vi "Download zip file.vi"(0 "client handle":T1, 5 "Artifactory ZIP Directory":string, 7 "Zip File":string, 9 "Save Path":path=path "C:/Automation/APLs", 11 "Error In":errorcluster) -> (4 "client handle out":T1, 8 "Output Path":path, 10 "file or folder exists?":bool, 15 "Error Out":errorcluster)   [LabVIEW 2016]
uses:
  <vilib>/httpClient/ClientHandle.ctl
  <vilib>/regexp/Match Regular Expression.xnode
  <vilib>/httpClient/LabVIEWHTTPClient.lvlib
  <vilib>/zip/NI_Unzip.lvlib
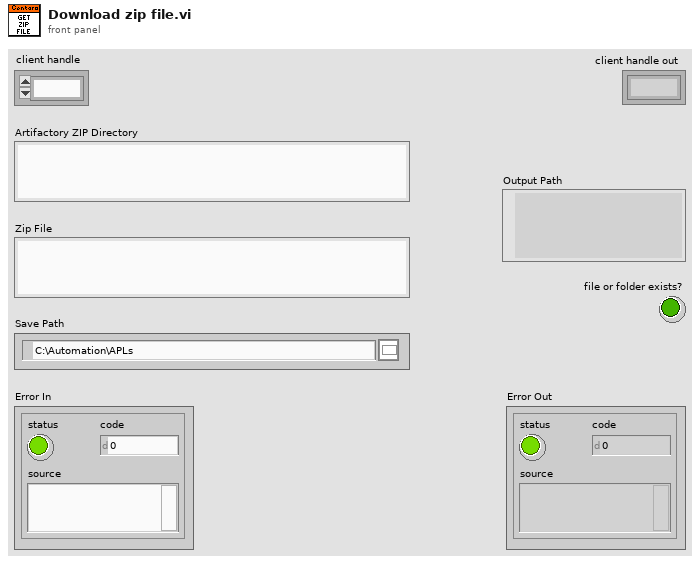
[diagram p1: front panel]
types:
  T1 = typedef "LabVIEWHTTPClient.lvlib/ClientHandle.ctl" = refnum<k1>
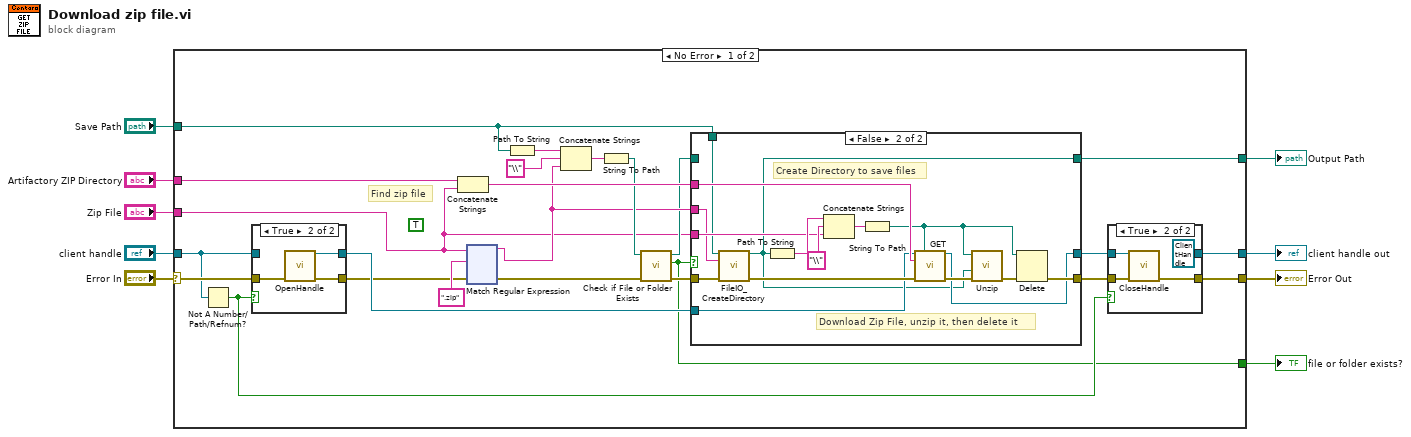
[diagram p0: block diagram]
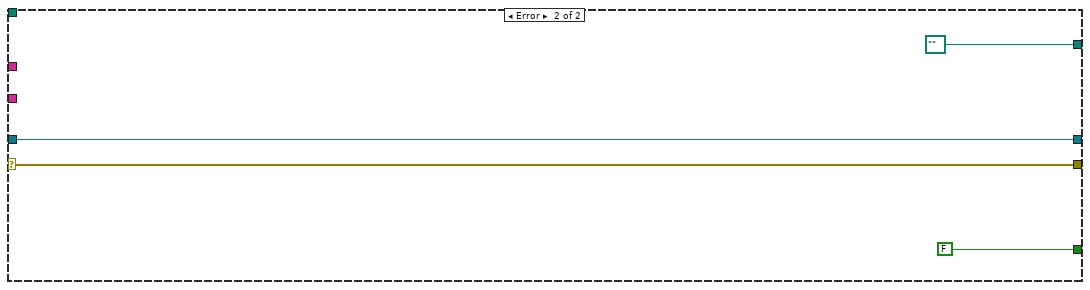
[diagram p5: hidden frame]
diagram:
  n1 = case shown="No Error" "Error In" {
    selector: "Error In" -> [w31 w181]
    tunnel: "client handle" -> [w24 w180]
    tunnel: [w33 w180] -> w8
    tunnel: [w32 w181] -> w7
    tunnel: "Artifactory ZIP Directory" -> [w28 _]
    tunnel: [w25 path ""] -> w4
    tunnel: "Save Path" -> [w21 _]
    tunnel: "Zip File" -> [w11 _]
    tunnel: [w13 FALSE ("file or folder exists?")] -> w1
    frame No Error {
      (unwired) TRUE ("multiline? (F)")
      # "Find zip file"
      n2 = Not A Number/Path/Refnum?(number/path/refnum=w24) -> (NaN/Path/Refnum?=w23:bool)
      n3 = case shown="True" w23 {
        tunnel: [w174 w177] -> w22
        tunnel: w24 -> [w174 _]
        tunnel: w31 -> [w173 w176]
        tunnel: [w173 w175] -> w10
        frame False {
        }
        frame True {
          n4 = call <vilib>:"OpenHandle.vi"("error in (no error)"=w176) -> ("client handle out"=w177:T1, "error out"=w175:errorcluster)  [unwired: 13 in]
        }
      }
      n5 = Concatenate Strings(w28, w11) -> (w29:string)
      n6 = xnode "Match Regular Expression"("input string"=w11, "regular expression"=".zip", "error in"=w10) -> ("before match"=w15:string, "error out"=w18:errorcluster)  [unwired: 3 in, 3 out]
      n7 = Path To String(path=w21) -> (string=w20:string)
      n8 = Concatenate Strings(w20, "\\" ("string"), w15) -> (w12:string)
      n9 = String To Path(string=w12) -> (path=w16:path)
      n10 = call <vilib>:"Check if File or Folder Exists.vi"("error in (no error)"=w18, "path"=w16) -> ("error out"=w17:errorcluster, "file or folder exists?"=w13:bool, "dup path"=w14:path)  [unwired: 7 in]
      n11 = case shown="False" w13 {
        tunnel: w11 -> [_ w48]
        tunnel: w15 -> [_ w47]
        tunnel: w17 -> [w36 w46]
        tunnel: w29 -> [_ w44]
        tunnel: [w36 w43] -> w27
        tunnel: [w35 w41] -> w26
        tunnel: w21 -> [_ w40]
        tunnel: [w34 w37] -> w25
        tunnel: w22 -> [w35 w38]
        tunnel: w14 -> [w34 _]
        frame True {
        }
        frame False {
          # "Create Directory to save files"
          # "Download Zip File, unzip it, then delete it"
          n12 = call "FileIO_CreateDirectory.vi"("Base Path"=w40, "Directory Name"=w47, "Error In"=w46) -> ("File Path Control"=w37:path, "Error Out"=w45:errorcluster)  [unwired: 11 in]
          n13 = Path To String(path=w37) -> (string=w52:string)
          n14 = Concatenate Strings(w52, "\\" ("string"), w48) -> (w50:string)
          n15 = String To Path(string=w50) -> (path=w39:path)
          n16 = call <vilib>:"GET.vi"("client handle"=w38, "output file"=w39, "url"=w44, "error in (no error)"=w45) -> ("client handle out"=w41:T1, "error out"=w42:errorcluster)  [unwired: 8 in, 2 out]
          n17 = call <vilib>:"Unzip.vi"("error in (no error)"=w42, "Target directory (same as Zip file if empty)"=w37, "Zip file"=w39) -> ("error out"=w51:errorcluster)  [unwired: 6 in, 2 out]
          n18 = Delete(path (use dialog)=w39, error in=w51) -> (error out=w43:errorcluster)  [unwired: 3 in, 2 out]
        }
      }
      n19 = case shown="True" w23 {
        tunnel: [w168 T1 refnum ("client handle out")] -> w33
        tunnel: w26 -> [w168 w170]
        tunnel: w27 -> [w167 w172]
        tunnel: [w167 w171] -> w32
        frame False {
        }
        frame True {
          n20 = call <vilib>:"CloseHandle.vi"("client handle"=w170, "error in (no error)"=w172) -> ("error out"=w171:errorcluster)  [unwired: 13 in]
        }
      }
    }
    frame Error {
    }
  }
  "Error Out" <- w7
  "Output Path" <- w4
  "client handle out" <- w8
  "file or folder exists?" <- w1
